vi "Experiment_treatment1_ArtemVer2_FastKG.vi"() -> ()   [LabVIEW 2018]
uses:
  <vilib>/Analysis/NI_AALBase.lvlib
  <vilib>/Analysis/1siggen.llb/Ramp Pattern by Samples.vi
  <vilib>/Utility/file.llb/Read From Spreadsheet File (DBL).vi
  dll_creation/x64/Release/test_dll_creation.dll
panel:
  in  "ratio_perm":dbl
  in  "length":i32=199847
  out "size(s)":i32[](array[numeric])=[199847, 4]
  out "Working time":dbl=2.45
  in  "Array":string[](array[string])=["Number", "MSE", "Eff. Deg. of Freedom", "Conf. interval size", "Nearest param 1", "Nearest param 2", "Nearest param 3", "Nearest param 4", "Math Exp of param 1", "Math Exp of param 2", "Math Exp of param 3", "Math Exp of param 4", "Stand Dev of param 1", "Stand Dev of param 2", "Stand Dev of param 3", "Stand Dev of param 4", "HPD Intercepts"]
  out "Clusters":i32=1307
  out "Tree built":i32=1
  out "k":dbl=4.721612219080669
  out "Stand Dev":dbl[](array[numeric])=[0.14906861116712494, 0.05810581607974299, 0.0031962555144778412, 11.46265609981548]
  out "Math Exp":dbl[](array[numeric])=[0.6778682211166033, 0.1513336118851721, 1.3771152122092714, 20.557420513696997]
  in  "Database type":u16(ring) items=["Random", "Regular", "Piecewise regular", "DiRect (not realized)"]
  out "MSE":dbl
  out "Nearest Params":sgl[](array[numeric])=[0.6691142, 0.11346816, 1.3706137, 46.785797]
  in  "Load":bool=TRUE
  in  "Params bounds":sgl[][](array[numeric])=[[0.5, 2.12], [0.1, 1.0], [1.37, 1.39], [0.0, 90.0]]
  in  "Database path":path=path "E:/OnEngFiles - science/test labview/4_add_cluster_lib/Plt_200k_h.db"
  in  "Angle bounds":i32[](array[numeric])=[10, 70]
  in  "Path to indicatrices":path=path "E:/OnEngFiles - science/test labview/4_add_cluster_lib/experiment_1000.txt"
  in  "How many to process":u16(ring)=1000 items=["All (889)"=889, "100"=100, "300"=300, "1000"=1000]
  in  "Launch":bool=TRUE
  in  "Tab Control":enum32{"Nearest Indicatrix"}(tab)
  out "XY Graph":cluster{"Y":dbl[], "Y":dbl[]}[](graph)=[{"Y"=[10.0, 11.0, 12.0, 13.0, 14.0, 15.0, 16.0, 17.0, 18.0, 19.0, 20.0, 21.0, 22.0, 23.0, 24.0, 25.0, 26.0, 27.0, 28.0, 29.0, 30.0, 31.0, 32.0, 33.0, 34.0, 35.0, 36.0, 37.0, 38.0, 39.0, 40.0, 41.0, 42.0, 43.0, 44.0, 45.0, 46.0, 47.0, 48.0, 49.0, 50.0, 51.0, 52.0, 53.0, 54.0, 55.0, 56.0, 57.0, 58.0, 59.0, 60.0], "Y"=[3.584928234374043e-05, 6.087175402032172e-05, 9.562049901976253e-05, 0.00014104691333700342, 0.00019757729815979622, 0.0002651135616544077, 0.00034308135664397625, 0.0004305081801215161, 0.0005261160539134097, 0.0006284168548823555, 0.0007358019994202503, 0.0008466213987461039, 0.000959249146877231, 0.001072135255465285, 0.0011838439896287526, 0.0012930801075181364, 0.0013987046879531642, 0.0014997423548416817, 0.0015953816629734523, 0.0016849702645666232, 0.0017680062781895245, 0.0018441270646478013, 0.0019130963996333134, 0.0019747908332749266, 0.0020291858490397796, 0.0020763422814356666, 0.0021163933237562708, 0.002149532352204729, 0.0021760017087887502, 0.0021960825196998424, 0.0022100855757161406, 0.0022183432638865374, 0.002221202512987111, 0.002219018696900437, 0.002212150428362565, 0.0022009551689452394, 0.0021857855784477988, 0.002166986527051351, 0.0021448926958249283, 0.0021198266948269017, 0.002092097632614167, 0.00206200007607233, 0.0020298133448228444, 0.001995801089834237, 0.001960211111111111, 0.0019232753743506287, 0.001885210191172391, 0.0018462165319028346, 0.001806480443909125, 0.0017661735521253483, 0.0017254536217018342]}, {"Y"=[10.0, 11.0, 12.0, 13.0, 14.0, 15.0, 16.0, 17.0, 18.0, 19.0, 20.0, 21.0, 22.0, 23.0, 24.0, 25.0, 26.0, 27.0, 28.0, 29.0, 30.0, 31.0, 32.0, 33.0, 34.0, 35.0, 36.0, 37.0, 38.0, 39.0, 40.0, 41.0, 42.0, 43.0, 44.0, 45.0, 46.0, 47.0, 48.0, 49.0, 50.0, 51.0, 52.0, 53.0, 54.0, 55.0, 56.0, 57.0, 58.0, 59.0, 60.0], "Y"=[0.0032144944874749623, 0.0032132298573099827, 0.0029659495363371217, 0.002712444976221678, 0.0026041146328709443, 0.0026259121642624654, 0.002644837766779372, 0.00252843040674818, 0.002242430201747389, 0.0018692780710884763, 0.0015507701572525703, 0.0014033129107546734, 0.0014598002632086123, 0.0016651567756611541, 0.0019170085087040311, 0.0021208737801508017, 0.0022290668182410028, 0.002248300373317722, 0.00222018160530276, 0.00219078906764674, 0.00218647057471567, 0.002205583659012032, 0.0022259928432159367, 0.002220926031811844, 0.00217379465770865, 0.0020852619171353236, 0.001970885484555106, 0.001852323331685977, 0.0017474430288977488, 0.0016641427256584055, 0.0016000347051028934, 0.0015469366635793708, 0.0014969545376869507, 0.0014467263688878807, 0.0013979689937462982, 0.0013547633161661095, 0.0013197453682908813, 0.0012916557375020025, 0.0012655875700386733, 0.0012355249800443844, 0.0011974685704525838, 0.0011512530107925744, 0.0011000865603667544, 0.0010482239528080827, 0.0009982067125814931, 0.0009492368672763391, 0.0008975231352131822, 0.0008383424657175091, 0.0007687260034128252, 0.0006895054184360893, 0.0006059307798655672]}]
  in  "Show graphs":bool
  in  "Calc ME and SD":bool=TRUE
  in  "Clasterization":bool=TRUE
  in  "Use built tree":bool
  out "Progress bar":u8(slide)=100 scale=0.0..100.0
  in  "output cluster":T1
  # "Database setup"
  # "Experiment setup"
  # "±"
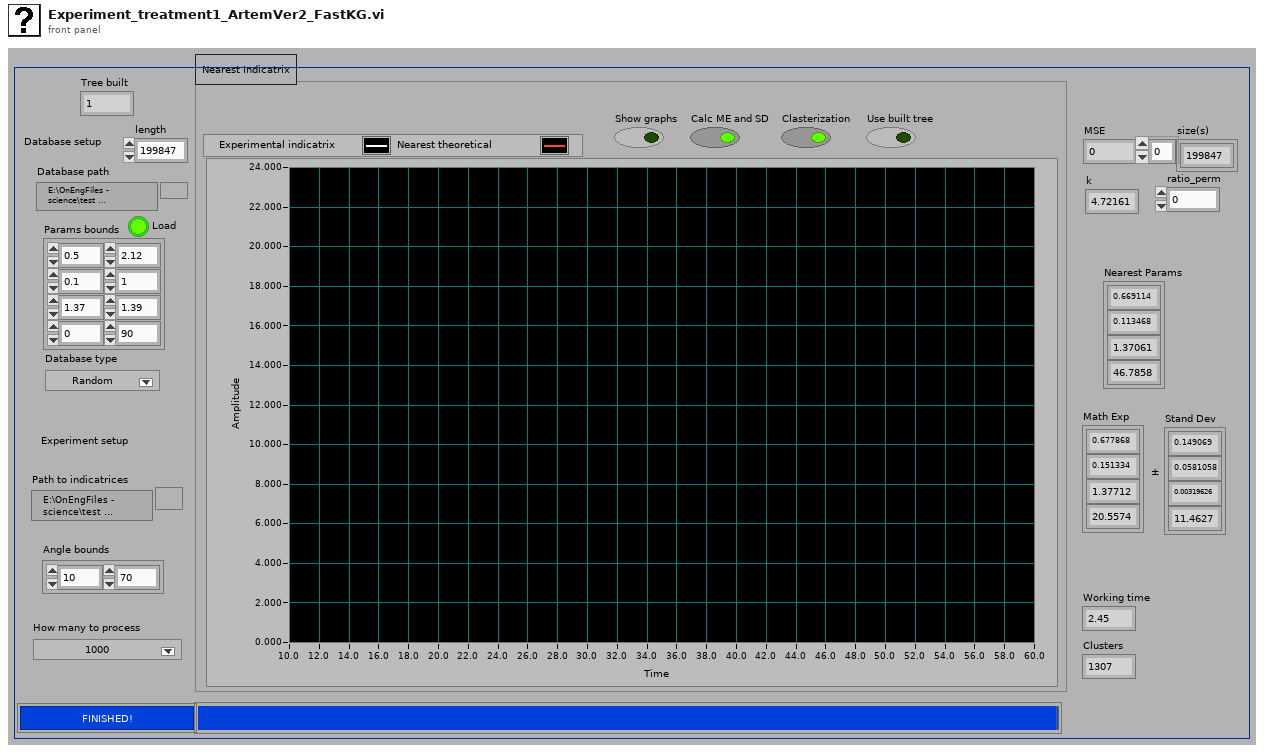
[diagram p1: front panel]
types:
  T1 = cluster{"Angles start":dbl, "Angles end":dbl, "Number of angles":i32, "Params bounds":sgl[][], "Params":sgl[][], "Indicatrices":sgl[][]}
  T2 = typedef "LVStringsAndValuesArrayTypeDef_U16.ctl" = cluster{"String":string, "Value":u16}[]
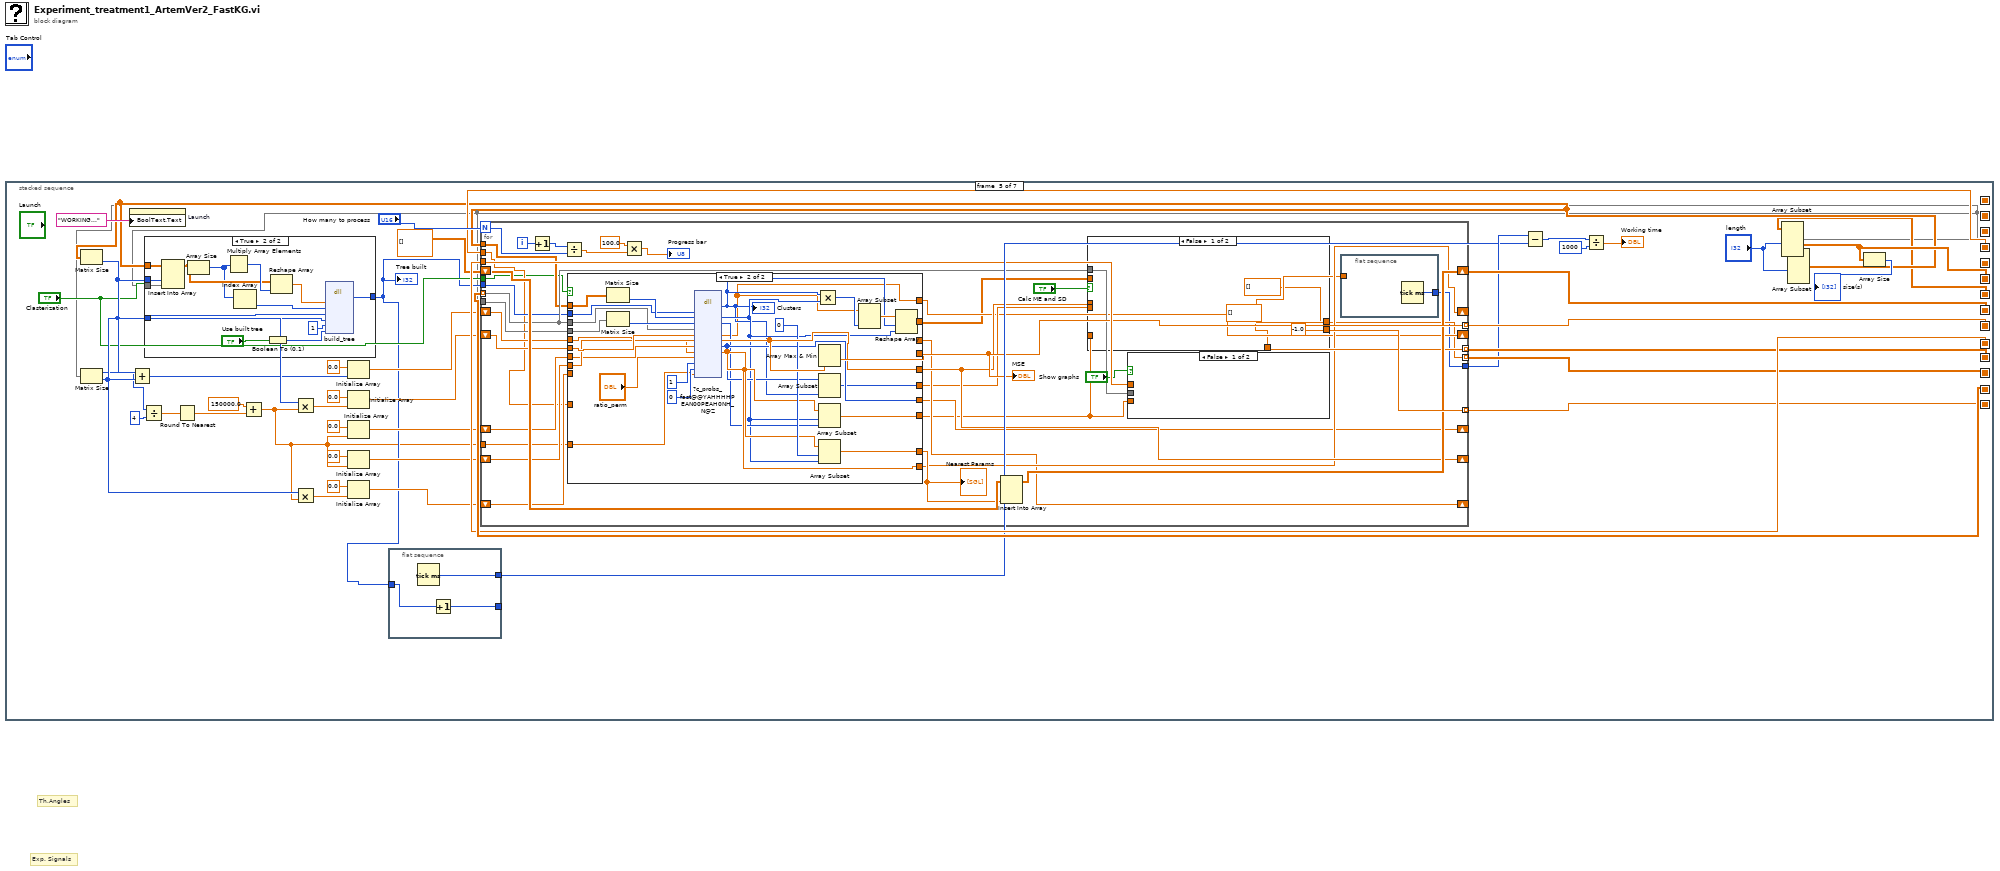
[diagram p0: block diagram]
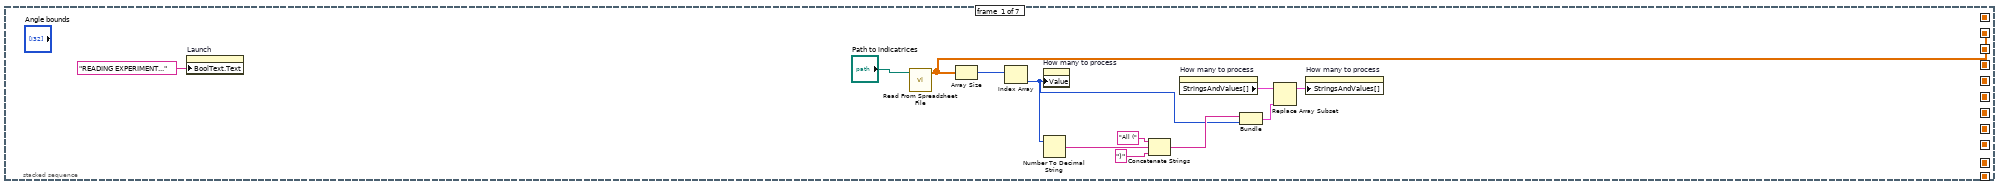
[diagram p2: hidden frame]
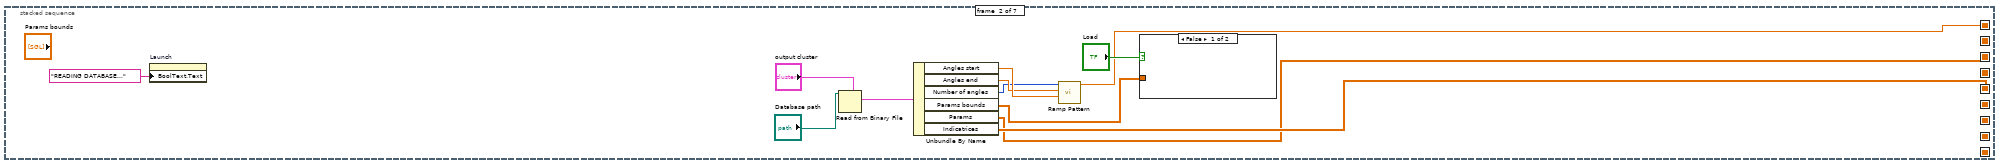
[diagram p3: hidden frame]
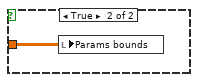
[diagram p4: hidden frame]
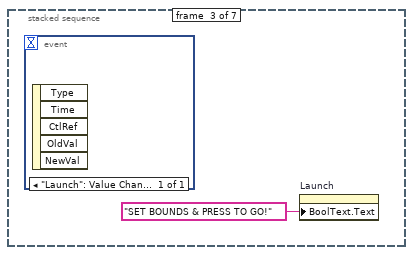
[diagram p5: hidden frame]
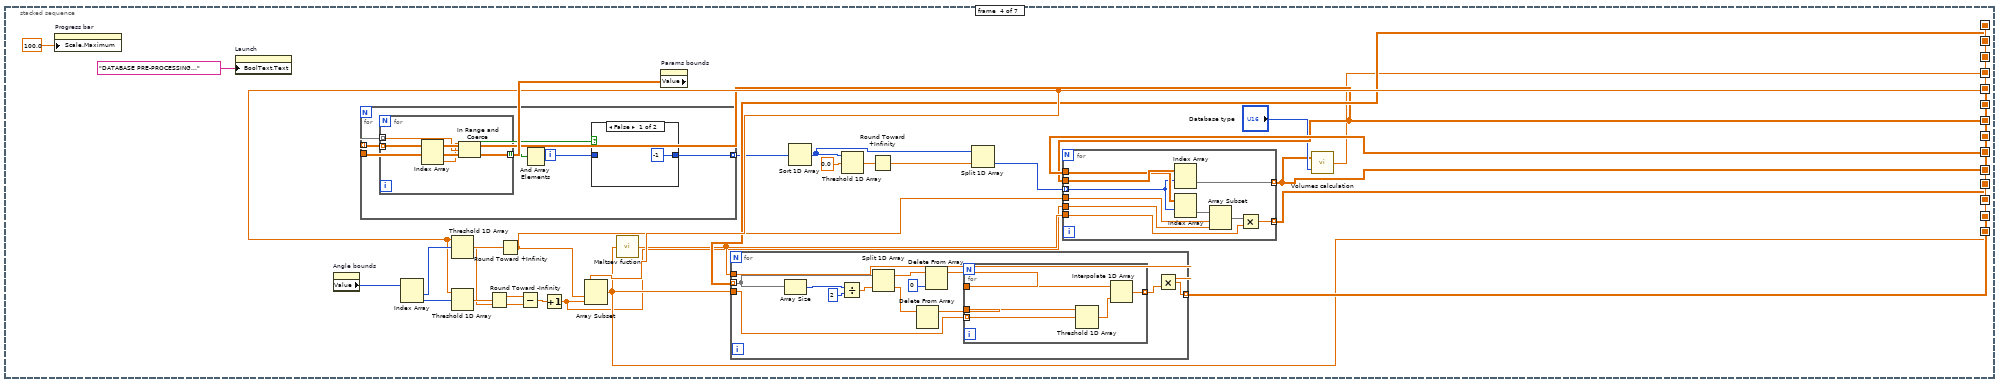
[diagram p6: hidden frame]
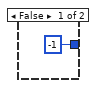
[diagram p8: hidden frame]
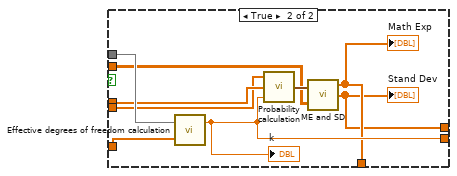
[diagram p9: hidden frame]
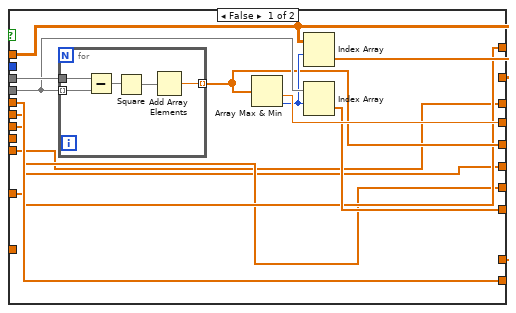
[diagram p10: hidden frame]
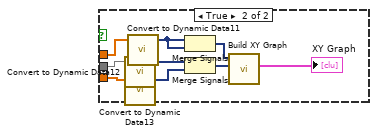
[diagram p11: hidden frame]
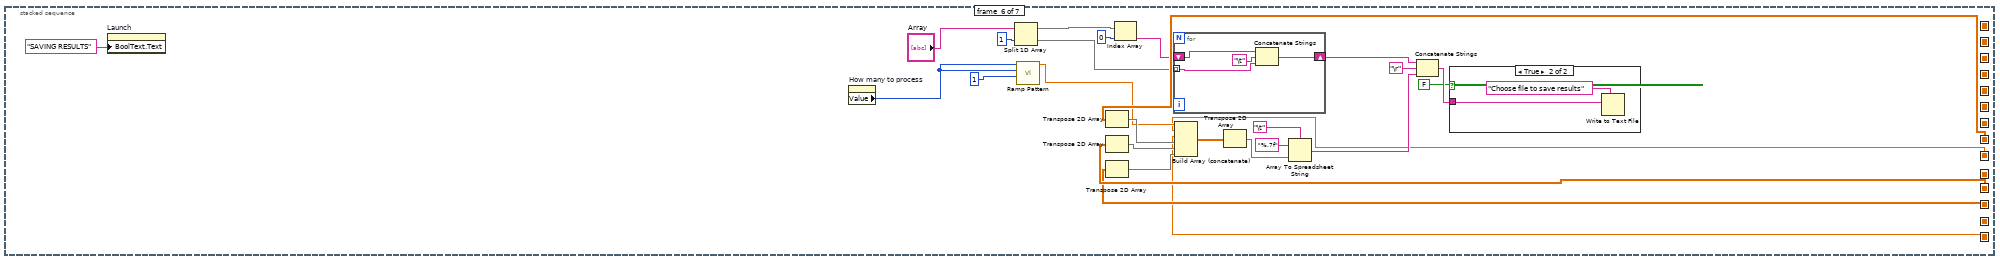
[diagram p12: hidden frame]
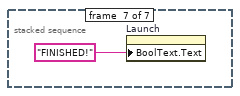
[diagram p14: hidden frame]
diagram:
  # "Th.Angles"
  # "Exp. Signals"
  n1 = stacked-sequence {
    seq-local: [_ w14 _ _ _ _ _] -> [_ _ _ w30 _ _ _]
    seq-local: [_ w21 _ _ _ _ _] -> [_ _ _ w42 _ _ _]
    seq-local: [w1 _ _ _ _ _ _] -> [_ _ _ w45 _ _ _]
    seq-local: [_ w19 _ _ _ _ _] -> [_ _ _ w49 _ _ _]
    seq-local: [_ _ _ w27 _ _ _] -> [_ _ _ _ w101 _ _]
    seq-local: [_ _ _ w41 _ _ _] -> [_ _ _ _ w99 _ _]
    seq-local: [_ _ _ w44 _ _ _] -> [_ _ _ _ w139 _ _]
    seq-local: [_ _ _ w43 _ _ _] -> [_ _ _ _ w138 _ _]
    seq-local: [_ _ _ w29 _ _ _] -> [_ _ _ _ w136 _ _]
    seq-local: [_ _ _ _ w134 _ _] -> [_ _ _ _ _ w289 _]
    seq-local: [_ _ _ _ w135 _ _] -> [_ _ _ _ _ w274 _]
    seq-local: [_ _ _ _ w133 _ _] -> [_ _ _ _ _ w288 _]
    seq-local: [_ _ _ _ w132 _ _] -> [_ _ _ _ _ w287 _]
    seq-local: [_ _ _ _ w131 _ _] -> [_ _ _ _ _ w272 _]
    frame #0 {
      n2 = property on="Launch" class="Bool (strict)"("BoolText.Text"="READING EXPERIMENT..." ("Boolean Text.Text")) -> ()  [unwired: 2 in, 2 out]
      n3 = call-poly <vilib>:"Read From Spreadsheet File.vi"("file path (dialog if empty)"="Path to indicatrices") -> ("all rows"=w1:dbl[][])  [unwired: 6 in, 4 out]
      n4 = Array Size(array=w1) -> (size(s)=w6:i32[])
      n5 = Index Array(array=w6) -> (element=w2:i32)  [unwired: 1 in]
      n6 = property on="How many to process" class="Ring (strict)"("Value"=w2) -> ()  [unwired: 2 in, 2 out]
      n7 = Number To Decimal String(number=w2) -> (decimal integer string=w3:string)  [unwired: 1 in]
      n8 = Concatenate Strings("All (" ("String"), w3, ")" ("String")) -> (w5:string)
      n9 = property on="How many to process" class="Ring (strict)"() -> ("StringsAndValues[]"=w10:T2)  [unwired: 2 in, 2 out]
      n10 = Bundle(w5, w2) -> (w8:cluster{string, i32})  [unwired: 1 in]
      n11 = Replace Array Subset(array=w10, new element=w8) -> (w11:T2)  [unwired: 1 in]
      n12 = property on="How many to process" class="Ring (strict)"("StringsAndValues[]"=w11) -> ()  [unwired: 2 in, 2 out]
    }
    frame #1 {
      n13 = property on="Launch" class="Bool (strict)"("BoolText.Text"="READING DATABASE..." ("Boolean Text.Text")) -> ()  [unwired: 2 in, 2 out]
      n14 = Read from Binary File(5:"output cluster", 11:"Database path") -> (2:w24:T1)  [unwired: 4 in, 3 out]
      n15 = Unbundle By Name(w24) -> ("Angles start"=w20:dbl, "Angles end"=w18:dbl, "Number of angles"=w17:i32, "Params bounds"=w16:sgl[][], "Params"=w14:sgl[][], "Indicatrices"=w21:sgl[][])
      n16 = call-poly <vilib>:"Ramp Pattern.vi"("start"=w20, "end"=w18, "samples"=w17) -> ("Ramp Pattern"=w19:dbl[])  [unwired: 7 in, 1 out]
      n17 = case shown="False" "Load" {
        tunnel: w16 -> [_ w25]
        frame False {
        }
        frame True {
          n18 = local write "Params bounds"(w25) -> ()
        }
      }
    }
    frame #2 {
      n19 = event shown="[0] \"Launch\": Value Change" {
        selector: _ -> [_]
        dyn-events: _ -> [_]
        timeout: _ -> [_]
        event "Launch": Value Change {
          n20 = event-data() -> ()  [unwired: 1 in, 5 out]
        }
      }
      n21 = property on="Launch" class="Bool (strict)"("BoolText.Text"="SET BOUNDS & PRESS TO GO!" ("Boolean Text.Text")) -> ()  [unwired: 2 in, 2 out]
    }
    frame #3 {
      n22 = property on="Progress bar" class="Slide (strict)"("Scale.Maximum"=100.0 ("Scale.Range:Maximum")) -> ()  [unwired: 2 in, 2 out]
      n23 = property on="Launch" class="Bool (strict)"("BoolText.Text"="DATABASE PRE-PROCESSING..." ("Boolean Text.Text")) -> ()  [unwired: 2 in, 2 out]
      n24 = property on="Angle bounds" class="Arr (strict)"() -> ("Value"=w53:i32[])  [unwired: 2 in, 2 out]
      n25 = Index Array(array=w53) -> (element #1=w52:i32, element #2=w46:i32)  [unwired: 2 in]
      n26 = Threshold 1D Array(2:w52, 3:w49) -> (0:w51:dbl)  [unwired: 1 in]
      n27 = Threshold 1D Array(2:w46, 3:w49) -> (0:w50:dbl)  [unwired: 1 in]
      n28 = Round Toward -Infinity(1:w50) -> (0:w48:dbl)
      n29 = Round Toward +Infinity(x=w51) -> (ceil(x): smallest int >= x=w38:dbl)
      n30 = Subtract(x=w48, y=w38) -> (x-y=w47:dbl)
      n31 = Increment(x=w47) -> (x+1=w39:dbl)
      n32 = Array Subset(array=w49, index=w38, length=w39) -> (w43:dbl[])
      n33 = call "Maltsev fuction.vi"("Angles"=w43) -> ("Maltsev fuction"=w40:dbl[])
      n34 = property on="Params bounds" class="Arr (strict)"() -> ("Value"=w54:sgl[][])  [unwired: 2 in, 2 out]
      n35 = for {
        tunnel: w30 -> [w87] mode=indexing
        tunnel: w54 -> [w89]
        tunnel: [w84] -> w37 mode=indexing
        i -> [w85]
        n36 = for {
          tunnel: w89 -> [w96] mode=indexing
          tunnel: w87 -> [w95] mode=indexing
          tunnel: [w92] -> w88 mode=indexing
          n37 = Index Array(array=w96) -> (element #1=w94:sgl, element #2=w93:sgl)  [unwired: 2 in]
          n38 = In Range and Coerce(upper limit=w93, x=w95, lower limit=w94) -> (In Range?=w92:bool)  [unwired: 1 out]
        }
        n39 = And Array Elements(Boolean array=w88) -> (logical AND=w86:bool)
        n40 = case shown="False" w86 {
          tunnel: w85 -> [_ w91]
          tunnel: [-1 w91] -> w84
          frame False {
          }
          frame True {
          }
        }
      }
      n41 = for {
        tunnel: w45 -> [w72] mode=indexing
        tunnel: w43 -> [w69]
        tunnel: w40 -> [w68]
        tunnel: [w66] -> w44 mode=indexing
        n42 = Array Size(array=w72) -> (size(s)=w76:i32)
        n43 = Divide(x=w76, y=2) -> (x/y=w75:dbl)
        n44 = Split 1D Array(array=w72, index=w75) -> (first subarray=w78:dbl[], second subarray=w77:dbl[])
        n45 = Delete From Array(array=w77) -> (array with subset deleted=w70:dbl[])  [unwired: 2 in, 1 out]
        n46 = Delete From Array(array=w78, index=0) -> (array with subset deleted=w71:dbl[])  [unwired: 1 in, 1 out]
        n47 = for {
          tunnel: w71 -> [w82]
          tunnel: w70 -> [w81]
          tunnel: w69 -> [w80] mode=indexing
          tunnel: [w79] -> w67 mode=indexing
          n48 = Threshold 1D Array(2:w80, 3:w81) -> (0:w83:dbl)  [unwired: 1 in]
          n49 = Interpolate 1D Array(1:w83, 2:w82) -> (0:w79:dbl)
        }
        n50 = Multiply(x=w68, y=w67) -> (x*y=w66:dbl[])
      }
      n51 = Sort 1D Array(array=w37) -> (sorted array=w33:i32[])
      n52 = Threshold 1D Array(2:0.0 ("threshold y"), 3:w33) -> (0:w35:dbl)  [unwired: 1 in]
      n53 = Round Toward +Infinity(x=w35) -> (ceil(x): smallest int >= x=w34:dbl)
      n54 = Split 1D Array(array=w33, index=w34) -> (second subarray=w32:i32[])  [unwired: 1 out]
      n55 = for {
        tunnel: w30 -> [w65]
        tunnel: w42 -> [w64]
        tunnel: [w63] -> w27 mode=indexing
        tunnel: [w60] -> w41 mode=indexing
        tunnel: w40 -> [w59]
        tunnel: w39 -> [w58]
        tunnel: w38 -> [w57]
        tunnel: w32 -> [w56] mode=indexing
        n56 = Index Array(array=w65, index (row)=w56) -> (element=w63:sgl[])  [unwired: 1 in]
        n57 = Index Array(array=w64, index (row)=w56) -> (element=w61:sgl[])  [unwired: 1 in]
        n58 = Array Subset(array=w61, index=w57, length=w58) -> (w62:sgl[])
        n59 = Multiply(x=w62, y=w59) -> (x*y=w60:dbl[])
      }
      n60 = call "Volumes calculation.vi"("Ring"="Database type", "Params"=w27) -> ("Volumes"=w29:sgl[])
    }
    frame #4 {
      n61 = property on="Launch" class="Bool (strict)"("BoolText.Text"="WORKING..." ("Boolean Text.Text")) -> ()  [unwired: 2 in, 2 out]
      n62 = flat-sequence {
        tunnel: [w144] -> w109
        tunnel: w104 -> [w143]
        tunnel: [w142] -> _
        frame #0 {
          n63 = Tick Count (ms)() -> (millisecond timer value=w144:u32)
          n64 = Increment(x=w143) -> (x+1=w142:i32)
        }
      }
      n65 = Array Subset(array=w99, length (row)="length") -> (w98:dbl[][])  [unwired: 3 in]
      n66 = Matrix Size(0:w98) -> (1:w114:i32, 2:w117:i32)
      n67 = Divide(x=w114, y=4) -> (x/y=w112:dbl)
      n68 = Round To Nearest(number=w112) -> (nearest integer value=w111:dbl)
      n69 = Add(x=150000.0 ("element"), y=w111) -> (x+y=w97:dbl)
      n70 = Multiply(x=w117, y=w97) -> (x*y=w118:dbl)
      n71 = Initialize Array(0.0 ("element"), w97) -> (w121:dbl[])
      n72 = Initialize Array(0.0 ("element"), w97) -> (w122:dbl[])
      n73 = Initialize Array(0.0 ("element"), w118) -> (w116:dbl[])
      n74 = Array Subset(array=w101, length (row)="length") -> (w100:sgl[][])  [unwired: 3 in]
      n75 = Matrix Size(0:w100) -> (2:w130:i32)  [unwired: 1 out]
      n76 = Add(x=w130, y=w117) -> (x+y=w129:i32)
      n77 = case shown="True" "Clasterization" {
        tunnel: w130 -> [_ w158]
        tunnel: w100 -> [_ w151]
        tunnel: w98 -> [_ w150]
        tunnel: [-1 ("return type") w149] -> w104
        tunnel: w117 -> [_ w148]
        frame False {
        }
        frame True {
          n78 = Insert Into Array(array=w151, index (col)=w158, new element=w150) -> (w153:sgl[][])  [unwired: 1 in]
          n79 = Array Size(array=w153) -> (size(s)=w152:i32[])
          n80 = Multiply Array Elements(1:w152) -> (0:w154:i32)
          n81 = Index Array(array=w152) -> (element=w156:i32)  [unwired: 1 in]
          n82 = Boolean To (0,1)(Boolean="Use built tree") -> (0, 1=w146:i16)
          n83 = Reshape Array(w153, w154) -> (w155:sgl[])
          n84 = dll-call lib="E:/OnEngFiles - science/test labview/4_add_cluster_lib/dll_creation/x64/Release/test_dll_creation.dll" fn="build_tree"("data"=w155, "number_points"=w156, "hiden_size"=w158, "mesured_size"=w148, "save"=1, "use_saved"=w146) -> ("return type"=w149:i32)  [unwired: 9 in, 2 out]
        }
      }
      "Tree built" <- w104
      n85 = Multiply(x=w130, y=w97) -> (x*y=w128:dbl)
      n86 = Initialize Array(0.0 ("element"), w129) -> (w120:dbl[])
      n87 = Initialize Array(0.0 ("element"), w128) -> (w123:dbl[])
      n88 = for {
        N: "How many to process" -> [w193]
        tunnel: w100 -> [w174]
        tunnel: w98 -> [w173]
        tunnel: w139 -> [w183] mode=indexing
        tunnel: w138 -> [w189]
        shift-right: [w185] -> w134
        shift-left: sgl[][] [] ("Params") -> [w186]
        tunnel: w136 -> [w162]
        tunnel: [w188] -> w135 mode=indexing
        tunnel: [w184] -> w133 mode=indexing
        tunnel: [w166] -> w132 mode=indexing
        tunnel: [w187] -> w131 mode=indexing
        shift-right: [w168] -> _
        shift-left: w123 -> [w181]
        shift-right: [w179] -> _
        shift-left: w122 -> [w163]
        shift-right: [w172] -> _
        shift-left: w121 -> [w180]
        shift-right: [w176] -> _
        shift-left: w120 -> [w182]
        tunnel: w104 -> [w178]
        shift-right: [w175] -> _
        shift-left: w116 -> [w164]
        tunnel: [w165] -> w110
        tunnel: "Clasterization" -> [w161]
        tunnel: w97 -> [w159]
        i -> [w194]
        n89 = Increment(x=w194) -> (x+1=w190:i32)
        n90 = Divide(x=w190, y=w193) -> (x/y=w195:dbl)
        n91 = case shown="True" w161 {
          tunnel: [w220 w255] -> w188
          tunnel: w183 -> [w221 w250]
          tunnel: w182 -> [w213 w229]
          tunnel: w181 -> [w212 w249]
          tunnel: w163 -> [_ w248]
          tunnel: w180 -> [w211 w247]
          tunnel: [w215 w246] -> w179
          tunnel: w178 -> [_ w245]
          tunnel: [w219 w243] -> w177
          tunnel: [w213 w242] -> w176
          tunnel: w164 -> [w210 _]
          tunnel: [w212 w230] -> w168
          tunnel: [w210 _] -> w175
          tunnel: w174 -> [w214 w241]
          tunnel: w173 -> [w218 w240]
          tunnel: [w211 w239] -> w172
          tunnel: [w209 w238] -> w171
          tunnel: [w216 w236] -> w169
          tunnel: [w214 w231] -> w167
          tunnel: w162 -> [w209 _]
          tunnel: w159 -> [_ w227]
          frame False {
            n92 = for {
              tunnel: w221 -> [w226]
              tunnel: w218 -> [w225] mode=indexing
              tunnel: [w223] -> w215 mode=indexing
              n93 = Subtract(x=w226, y=w225) -> (x-y=w222:dbl[])
              n94 = Square(x=w222) -> (x^2=w224:dbl[])
              n95 = Add Array Elements(numeric array=w224) -> (sum=w223:dbl)
            }
            n96 = Array Max & Min(array=w215) -> (min value=w220:dbl, min index (indices)=w217:i32)  [unwired: 2 out]
            n97 = Index Array(array=w214, index (row)=w217) -> (element=w219:sgl[])  [unwired: 1 in]
            n98 = Index Array(array=w218, index (row)=w217) -> (element=w216:dbl[])  [unwired: 1 in]
          }
          frame True {
            n99 = Matrix Size(0:w241) -> (2:w254:i32)  [unwired: 1 out]
            n100 = Matrix Size(0:w240) -> (2:w253:i32)  [unwired: 1 out]
            n101 = dll-call lib="E:/OnEngFiles - science/test labview/4_add_cluster_lib/dll_creation/x64/Release/test_dll_creation.dll" fn="?c_probs_fast@@YAHHHHPEAN00PEAH0NH_N@Z"("number_points"=w245, "hiden_size"=w254, "mesured_size"=w253, "measure"=w250, "centers"=w249, "dist_s"=w248, "weights"=w247, "closest"=w229, "ratio_perm"="ratio_perm", "is_build_tree"=1, "load"=i8 0, "max_clust_num"=w227) -> ("return type"=w232:i32, "hiden_size"=w233:i32, "mesured_size"=w237:i32, "centers"=w230:dbl[], "dist_s"=w246:dbl[], "weights"=w239:i32[], "closest"=w242:dbl[])  [unwired: 9 in, 2 out]
            "Clusters" <- w232
            n102 = Multiply(x=w232, y=w233) -> (x*y=w235:i32)
            n103 = Array Max & Min(array=w246) -> (min value=w255:dbl)  [unwired: 3 out]
            n104 = Array Subset(array=w239, length=w232) -> (w238:i32[])  [unwired: 1 in]
            n105 = Array Subset(array=w242, index=w233, length=w237) -> (w236:dbl[])
            n106 = Array Subset(array=w242, index=0, length=w233) -> (w243:dbl[])
            n107 = Array Subset(array=w230, length=w235) -> (w234:dbl[])  [unwired: 1 in]
            n108 = Reshape Array(w234, w232, w233) -> (w231:dbl[][])
          }
        }
        "Nearest Params" <- w177
        "MSE" <- w188
        n109 = Multiply(x=100.0, y=w195) -> (x*y=→"Progress bar":dbl)
        n110 = Insert Into Array(array=w186, new element=w177) -> (w185:sgl[][])  [unwired: 2 in]
        n111 = case shown="False" "Calc ME and SD" {
          tunnel: [-1.0 ("effective degrees of freedom") w206] -> w187
          tunnel: [dbl[] [] ("ME") w205] -> w184
          tunnel: w183 -> [_ w204]
          tunnel: w179 -> [_ w203]
          tunnel: w171 -> [_ w202]
          tunnel: w169 -> [_ w201]
          tunnel: w167 -> [_ w200]
          tunnel: [dbl[] [] ("SD") w199] -> w166
          frame False {
          }
          frame True {
            n112 = call "Effective degrees of freedom calculation.vi"("nearest theoretical function from database"=w201, "experimental function"=w204) -> ("effective degrees of freedom"=w206:dbl)  [unwired: 1 out]
            "k" <- w206
            n113 = call "Probability calculation.vi"("effective degrees of freedom"=w206, "MSE array"=w203, "Volumes"=w202) -> ("Sorted Probabilities"=w207:cluster{dbl, dbl, i32}[])
            n114 = call "ME and SD.vi"("Array"=w200, "Sorted Probabilities"=w207) -> ("SD"=w199:dbl[], "ME"=w205:dbl[])  [unwired: 1 in]
            "Math Exp" <- w205
            "Stand Dev" <- w199
          }
        }
        n115 = case shown="False" "Show graphs" {
          tunnel: w189 -> [_ w258]
          tunnel: w183 -> [_ w259]
          tunnel: w169 -> [_ w257]
          frame False {
          }
          frame True {
            n116 = call "Convert to Dynamic Data12"("Array"=w259) -> ("Dynamic Data Type"=w262:dynamicdata)  [unwired: 3 in]
            n117 = call "Convert to Dynamic Data13"("Array"=w257) -> ("Dynamic Data Type"=w256:dynamicdata)  [unwired: 3 in]
            n118 = call "Convert to Dynamic Data11"("Array"=w258) -> ("Dynamic Data Type"=w260:dynamicdata)  [unwired: 3 in]
            n119 = Merge Signals(w260, w260) -> (w261:dynamicdata)
            n120 = Merge Signals(w262, w256) -> (w263:dynamicdata)
            n121 = call "Build XY Graph"("Y Input"=w263, "X Input"=w261) -> ("XY Graph"=→"XY Graph":cluster{"Y":dbl[], "Y":dbl[]}[])  [unwired: 8 in, 1 out]
          }
        }
        n122 = flat-sequence {
          tunnel: w166 -> [_]
          tunnel: [w208] -> w165
          frame #0 {
            n123 = Tick Count (ms)() -> (millisecond timer value=w208:u32)
          }
        }
      }
      n124 = Subtract(x=w110, y=w109) -> (x-y=w107:u32)
      n125 = Divide(x=w107, y=u32 1000) -> (x/y=→"Working time":dbl)
      n126 = Array Size(array=w101) -> (size(s)=→"size(s)":i32[])
    }
    frame #5 {
      n127 = property on="Launch" class="Bool (strict)"("BoolText.Text"="SAVING RESULTS" ("Boolean Text.Text")) -> ()  [unwired: 2 in, 2 out]
      n128 = property on="How many to process" class="Ring (strict)"() -> ("Value"=w286:u16)  [unwired: 2 in, 2 out]
      n129 = Split 1D Array(array="Array", index=1) -> (first subarray=w268:string[], second subarray=w269:string[])
      n130 = call-poly <vilib>:"Ramp Pattern.vi"("start"=1, "end"=w286, "samples"=w286) -> ("Ramp Pattern"=w275:dbl[])  [unwired: 7 in, 1 out]
      n131 = Transpose 2D Array(2D array=w289) -> (transposed array=w285:sgl[][])
      n132 = Transpose 2D Array(2D array=w288) -> (transposed array=w284:dbl[][])
      n133 = Transpose 2D Array(2D array=w287) -> (transposed array=w283:dbl[][])
      n134 = Index Array(array=w268, index=0) -> (element=w266:string)
      n135 = for {
        tunnel: w269 -> [w295] mode=indexing
        shift-right: [w294] -> w273
        shift-left: w266 -> [w297]
        n136 = Concatenate Strings(w297, "\t", w295) -> (w294:string)
      }
      n137 = Build Array (concatenate)(w275, w274, w272, w285, w284, w283) -> (w280:dbl[][])
      n138 = Transpose 2D Array(2D array=w280) -> (transposed array=w279:dbl[][])
      n139 = Array To Spreadsheet String(delimiter (Tab)="\t", array=w279, 3:"%.7f" ("format (%.3f)")) -> (spreadsheet string=w282:string)
      n140 = Concatenate Strings(w273, "\r", w282) -> (w281:string)
      n141 = case shown="True" FALSE {
        tunnel: w281 -> [_ w293]
        frame False {
        }
        frame True {
          n142 = Write to Text File(prompt (Choose or enter file path)="Choose file to save results", text=w293) -> ()  [unwired: 2 in, 3 out]
        }
      }
    }
    frame #6 {
      n143 = property on="Launch" class="Bool (strict)"("BoolText.Text"="FINISHED!" ("Boolean Text.Text")) -> ()  [unwired: 2 in, 2 out]
    }
  }
